vi "PrintScreen.vi"(0 "Take a screenshot":bool) -> ()   [LabVIEW 2014]
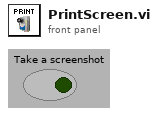
[diagram p1: front panel]
types:
  T1 = typedef "imagedata.ctl" = cluster{"image type":i32, "image depth":i32, "image":u8[], "mask":u8[], "colors":u32[], "Rectangle":cluster{"left":i16, "top":i16, "right":i16, "bottom":i16}}
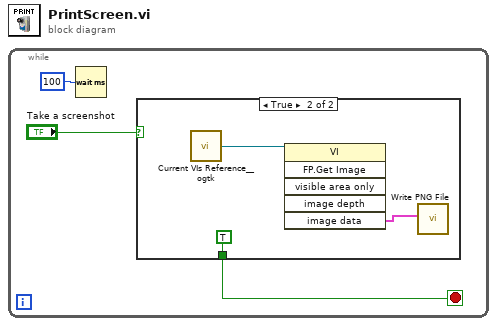
[diagram p0: block diagram]
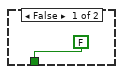
[diagram p2: hidden frame]
diagram:
  n1 = while {
    stop <- w1 stop-if-true
    n2 = Wait (ms)(milliseconds to wait=u32 100) -> ()  [unwired: 1 out]
    n3 = case shown="True" "Take a screenshot" {
      tunnel: [FALSE TRUE] -> w1
      frame False {
      }
      frame True {
        n4 = call <userlib>:"Current VIs Reference__ogtk.vi"() -> ("Current VI's reference"=w7:refnum<vi>)  [unwired: 5 in]
        n5 = invoke class="VI" method="FP.Get Image"(reference=w7) -> ("image data"=w5:T1)  [unwired: 5 in, 5 out]
        n6 = call <vilib>:"Write PNG File.vi"("image data"=w5) -> ()  [unwired: 9 in, 2 out]
      }
    }
  }
